vi "Set LabVIEW Parameters from Database.vi"(0 "Measurement Interface in":refnum<class "Measurement Interface.lvclass">, 5 "Step In":refnum<k7>, 7 "Dictionary Keys":string[](array[string]), 9 "LabVIEW Parameter Mapping":string[](array[string]), 11 "error in (no error)":errorcluster) -> (4 "Measurement Interface out":refnum<class "Measurement Interface.lvclass">, 6 "Step Out":refnum<k7>, 15 "error out":errorcluster)   [LabVIEW 2016, in "Measurement Interface.lvlib" / "Measurement Interface.lvclass"]
uses:
  Measurement Interface.lvclass
  Measurement Interface.lvclass/Measurement Interface.ctl
  Measurement Parameters/Read Measurement Parameters.vi
  Plugins/String Database.lvlibp/String Database.lvclass
  Plugins/TestStand API Tools (TSAT).lvlibp/Step Actions/TSAT Step Actions.lvlib
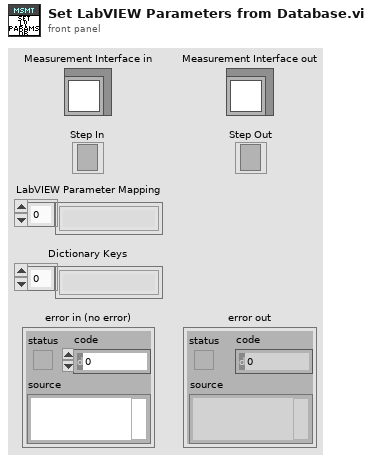
[diagram p1: front panel]
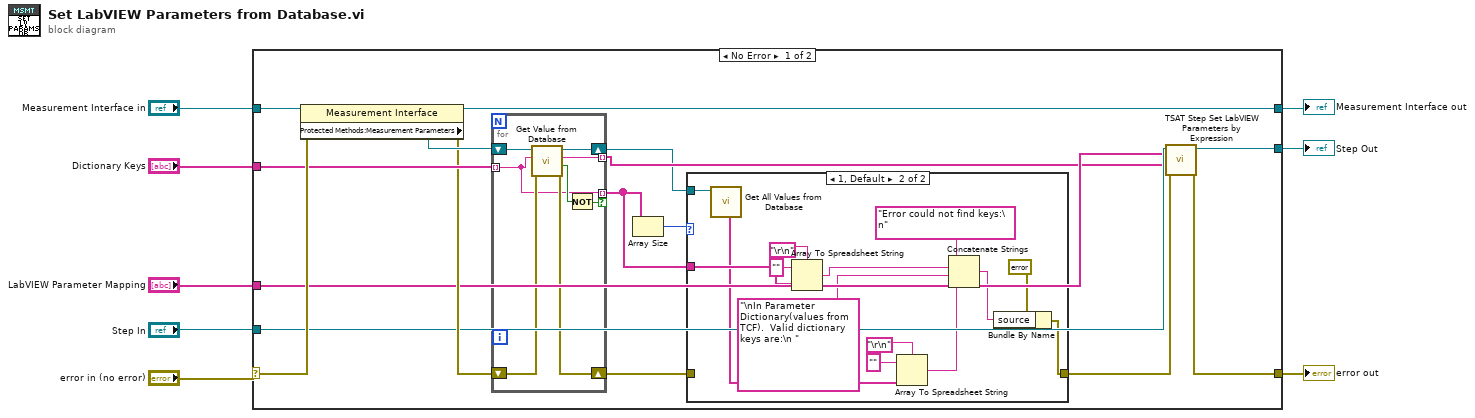
[diagram p0: block diagram]
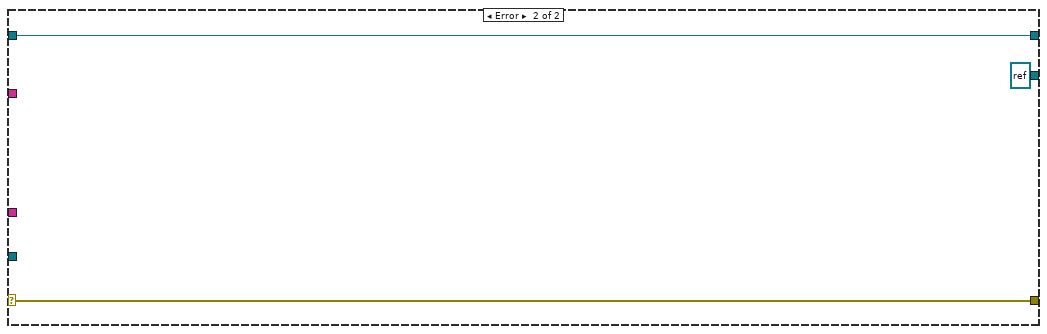
[diagram p3: hidden frame]
diagram:
  n1 = case shown="No Error" "error in (no error)" {
    selector: "error in (no error)" -> [w24 w50]
    tunnel: [w23 w50] -> w1
    tunnel: [w18 w49] -> w2
    tunnel: "Measurement Interface in" -> [w22 w49]
    tunnel: "LabVIEW Parameter Mapping" -> [w15 _]
    tunnel: "Dictionary Keys" -> [w20 _]
    tunnel: "Step In" -> [w17 _]
    tunnel: [w16 refnum<k7> refnum ("Step Out")] -> w5
    frame No Error {
      n2 = property class="Measurement Interface"(reference=w22, error in=w24) -> (reference out=w18:refnum<class "Measurement Interface.lvclass">, error out=w19:errorcluster, "Protected Methods:Measurement Parameters"=w21:refnum<class "String Database.lvclass">)
      n3 = for {
        shift-right: [w46] -> w9
        shift-left: w21 -> [w47]
        tunnel: [w43] -> w14 mode=indexing
        tunnel: w20 -> [w40] mode=indexing
        shift-right: [w45] -> w11
        shift-left: w19 -> [w44]
        tunnel: [w40] -> w12 mode=indexing if=w42
        n4 = call "Get Value from Database.vi"("error in (no error)"=w44, "Entry Name"=w40, "Message in"=w47) -> ("error out"=w45:errorcluster, "Entry Found"=w41:bool, "Entry Value"=w43:string, "Message out"=w46:refnum<class "String Database.lvclass">)  [unwired: 5 in]
        n5 = Not(x=w41) -> (.not. x?=w42:bool)
      }
      n6 = Array Size(array=w12) -> (size(s)=w13:i32)
      n7 = case shown="1, Default" w13 {
        tunnel: w12 -> [_ w36]
        tunnel: w11 -> [w25 _]
        tunnel: [w25 w38] -> w10
        tunnel: w9 -> [_ w30]
        frame 0 {
        }
        frame 1, Default {
          n8 = call "Get All Values from Database.vi"("String Database in"=w30) -> ("Names"=w26:string[])  [unwired: 7 in, 3 out]
          n9 = Array To Spreadsheet String(delimiter (Tab)="\r\n", array=w36, 3:"" ("format string")) -> (spreadsheet string=w33:string)
          n10 = Array To Spreadsheet String(delimiter (Tab)="\r\n", array=w26, 3:"" ("format string")) -> (spreadsheet string=w27:string)
          n11 = Concatenate Strings("Error could not find keys:\n", w33, "\nIn Parameter Dictionary(values from TCF).  Valid dictionary keys are:\n " ("string"), w27) -> (w37:string)
          n12 = Bundle By Name(cluster=errorcluster {"status"=TRUE, "code"=5601, "source"=""} ("error constant"), "source"=w37) -> (w38:errorcluster)
        }
      }
      n13 = call "TSAT Step Set LabVIEW Parameters by Expression.vi"("Error In"=w10, "Value Expressions"=w14, "Parameters to Set"=w15, "Step In"=w17) -> ("Error Out"=w23:errorcluster, "Step Out"=w16:refnum<k7>)  [unwired: 6 in]
    }
    frame Error {
    }
  }
  "error out" <- w1
  "Measurement Interface out" <- w2
  "Step Out" <- w5
